vi "Main.vi"(11 "Module Admin":refnum<class "Delacor_lib_QMH_Module Admin.lvclass">) -> ()   [LabVIEW 2020, in "GUI.lvlib"]
doc: "This template is based off of the Queued Message Handler design pattern and the Queued Message Handler project template that ships with LabVIEW.\n\nThe main difference is that the queue is private to this module and communication between modules is performed via Broadcast and Request events.\n\nRequest events are wrapped in public API methods and are handled in the Event Handling Loop (EHL) of this VI. Any module can register for Broadcast events sent by this module. The EHL generates messages based on user interface actions.\n\nThe Message Handling Loop (MHL) processes messages generated by the EHL, or by other messages. The messages are string values, so new messages can be added easily to the Message Cases case structure in the MHL. Each message cluster can also provide an optional value for Message Data, which is a variant that can be converted to whatever message-specific data is required.\n_____\nBased on DQMH Project Template 6.1.0.94."
uses:
  GUI.lvlib
  <vilib>/Delacor/Delacor QMH/Libraries/Module Admin_class/Delacor_lib_QMH_Module Admin.lvclass
  <vilib>/Delacor/Delacor QMH/Libraries/Message Queue_class/Delacor_lib_QMH_Message Queue.lvclass/Delacor_lib_QMH_Message Queue.ctl
  <vilib>/Delacor/Delacor QMH/Libraries/Module Admin_class/Delacor_lib_QMH_Module Admin.lvclass/Delacor_lib_QMH_Module Admin.ctl
  <vilib>/ErrorRing/Error Ring.xnode
  <vilib>/Delacor/Delacor QMH/Libraries/Message Queue_class/Delacor_lib_QMH_Message Queue.lvclass
  Module Data--cluster.ctl
  <vilib>/Utility/miscctls.llb/LVPointTypeDef.ctl
  <vilib>/Delacor/Delacor QMH/Libraries/Message Queue_class/Delacor_lib_QMH_Enqueue Message (Single).vi
  Stop Argument--cluster.ctl
  NI DAQ/NI DAQ.lvlib
  Support/Motor parameters.ctl
  Start motor Argument--cluster.ctl
  NI DAQ/Support/Task list.ctl
  NI DAQ/Support/Continuous aquisition params.ctl
  FGV states.ctl
  Configuration/Configuration.lvlib
  Configuration/Config data.ctl
  Stop conditions.ctl
  TDS1002 Oscilloscope/TDS1002 Oscilloscope.lvlib
  Support/Channel configuration--cluster.ctl
  TDS1002 Oscilloscope/Trigger config--cluster.ctl
  Support/Motor move data.ctl
  <vilib>/Delacor/Delacor QMH/Libraries/Message Queue_class/Delacor_lib_QMH_Enqueue Message (Array).vi
  <vilib>/Utility/error.llb/Error Cluster From Error Code.vi
  Support/Stop button.ctl
  Support/Home button.ctl
  Support/Move motor.ctl
  Support/Exit button.ctl
  Support/Configure button.ctl
panel:
  out "Homing?":bool
  in  "Pasos por medición":i32=50
  out "XY Graph":cluster{"X":dbl, "Y":dbl}[](graph)
  out "Lectura del sensor":dbl format="%#_gV"
  in  "Emergency stop":T1
  in  "stop":T2
  out "current position":dbl caption="Posición actual" format="%0.4f mm"
  in  "Home Button":T3
  in  "Configure":T4
  in  "Parámetros del motor":T5={"Dirección"=enum."Avance", "Tipo"=enum."Simple", "Velocidad (RPM)"=5.0, "Cantidad de pasos"=100} {"Cantidad de pasos" min=0 max=16000 step=1; "Velocidad (RPM)" min=1.0 max=100.0 step=1.0}
  in  "Stop motor":bool
  in  "Move motor":T6
  out "error out":errorcluster
  out "Status":string caption="Estado del sistema"
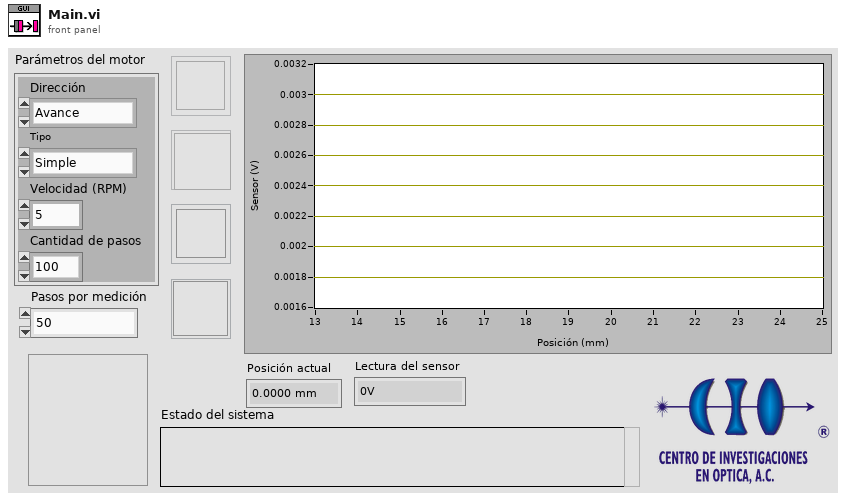
[diagram p1: front panel]
types:
  T1 = typedef "Stop button.ctl" = bool
  T2 = typedef "Exit button.ctl" = bool
  T3 = typedef "Home button.ctl" = bool
  T4 = typedef "Configure button.ctl" = bool
  T5 = cluster{"Dirección":enum16{"Avance", "Retroceso"}, "Tipo":enum16{"Simple", "Medio paso"}, "Velocidad (RPM)":dbl, "Cantidad de pasos":i32}
  T6 = typedef "Move motor.ctl" = bool
  T7 = typedef "GUI.lvlib/Module Data--cluster.ctl" = cluster{"Status":string, "DAQ mod ID":i32, "OSC mod ID":i32, "Config data":T8}
  T8 = typedef "Configuration.lvlib/Config data.ctl" = cluster{"Arduino":string, "Steps per rev":dbl, "Config path":path, "Pitch":dbl, "Osciloscopio":refnum<visa-resource-name>}
  T9 = typedef "NI DAQ.lvlib/Broadcast Events--cluster.ctl" = cluster{"Module Did Init":refnum<user-event>, "Status Updated":refnum<user-event>, "Error Reported":refnum<user-event>, "Module Did Stop":refnum<user-event>, "Update Module Execution Status":refnum<user-event>, "Digital data acquired":refnum<user-event>, "Device connected":refnum<user-event>, "Connection failed":refnum<user-event>, "Analog data acquired":refnum<user-event>, "Tasks started":refnum<user-event>}
  T10 = typedef "Configuration.lvlib/Broadcast Events--cluster.ctl" = cluster{"Module Did Init":refnum<user-event>, "Status Updated":refnum<user-event>, "Error Reported":refnum<user-event>, "Module Did Stop":refnum<user-event>, "Update Module Execution Status":refnum<user-event>}
  T11 = typedef "GUI.lvlib/Broadcast Events--cluster.ctl" = cluster{"Module Did Init":refnum<user-event>, "Status Updated":refnum<user-event>, "Error Reported":refnum<user-event>, "Module Did Stop":refnum<user-event>, "Update Module Execution Status":refnum<user-event>, "Motor stopped":refnum<user-event>}
  T12 = typedef "TDS1002 Oscilloscope.lvlib/Broadcast Events--cluster.ctl" = cluster{"Module Did Init":refnum<user-event>, "Status Updated":refnum<user-event>, "Error Reported":refnum<user-event>, "Module Did Stop":refnum<user-event>, "Update Module Execution Status":refnum<user-event>, "Helper Loop Status Updated":refnum<user-event>, "Device connected":refnum<user-event>, "Device disconnected":refnum<user-event>, "Data acquired":refnum<user-event>, "Configuration applied":refnum<user-event>}
  T13 = typedef "GUI.lvlib/Request Events--cluster.ctl" = cluster{"Stop Module":refnum<user-event>, "Show Panel":refnum<user-event>, "Hide Panel":refnum<user-event>, "Get Module Execution Status":refnum<user-event>, "Show Diagram":refnum<user-event>, "Start motor":refnum<user-event>, "Move motor":refnum<user-event>, "Stop motor":refnum<user-event>}
  T14 = typedef "Motor move data.ctl" = cluster{"current position":dbl, "Sensor reading (V)":dbl, "Home?":bool, "Steps taken":i32, "Graph data":cluster{"current position out":dbl, "Sensor reading":dbl}[], "Timeout":i32}
  T15 = typedef "GUI.lvlib/Stop conditions.ctl" = enum16{"Finish", "End-stop", "Manual"}
  T16 = cluster{"current position out":dbl, "Sensor reading":dbl}[]
  T17 = enum8{"Enabled", "Disabled", "Disabled and Grayed Out"}
  T18 = typedef "GUI.lvlib/FGV states.ctl" = enum16{"Read", "Full step", "Half step", "Release", "Reset"}
  T19 = typedef "LVPointTypeDef.ctl" = cluster{"Horizontal":i16, "Vertical":i16}
  T20 = enum32{"Invalid", "Standard", "Closed", "Hidden", "Minimized", "Maximized"}
  T21 = enum16{"All", "DO task", "DI task", "AO task", "AI task"}
  T22 = typedef "GUI.lvlib/Start motor Argument--cluster.ctl" = cluster{"Motor params":T23}
  T23 = typedef "GUI.lvlib/Motor parameters.ctl" = cluster{"Dirección":enum16{"Avance", "Retroceso"}, "Tipo":enum16{"Simple", "Medio paso"}, "Velocidad (RPM)":dbl, "Cantidad de pasos":i32, "Avance (mm)":dbl, "Pasos por rev":dbl, "Paso del tonillo":dbl}
  T24 = typedef "NI DAQ.lvlib/Task list.ctl" = enum16{"All", "DO task", "DI task", "AO task", "AI task"}
  T25 = typedef "NI DAQ.lvlib/Continuous aquisition params.ctl" = cluster{"Module ID":i32, "Task list":T24, "Timeout":i32, "Acq type":enum16{"Single", "Multiple"}, "Data in":variant, "DAQmx Task":refnum<k21>, "N samples":i32}
  T26 = typedef "GUI.lvlib/Stop Argument--cluster.ctl" = cluster{"Origin":string, "Exit via Stop Module Req?":bool, "Wait for Module to stop?":bool}
  T27 = enum32{"invalid lock state", "Not Locked", "Locked (No Password)", "Password-protected"}
  T28 = cluster{"current position":dbl, "Sensor reading (V)":dbl}
  T29 = cluster{"current position":dbl, "Sensor reading (V)":dbl}[]
  T30 = typedef "TDS1002 Oscilloscope.lvlib/Trigger config--cluster.ctl" = cluster{"Trigger Source":i32, "Trigger Mode":i32, "Trigger Slope":i32, "Trigger Coupling":i32, "Trigger Level":dbl}
  T31 = typedef "TDS1002 Oscilloscope.lvlib/Channel configuration--cluster.ctl" = cluster{"Acquisition Type":i32, "Averaged Waveforms":i32, "Channel":i32, "Probe Attenuation":i32, "Timebase":dbl}
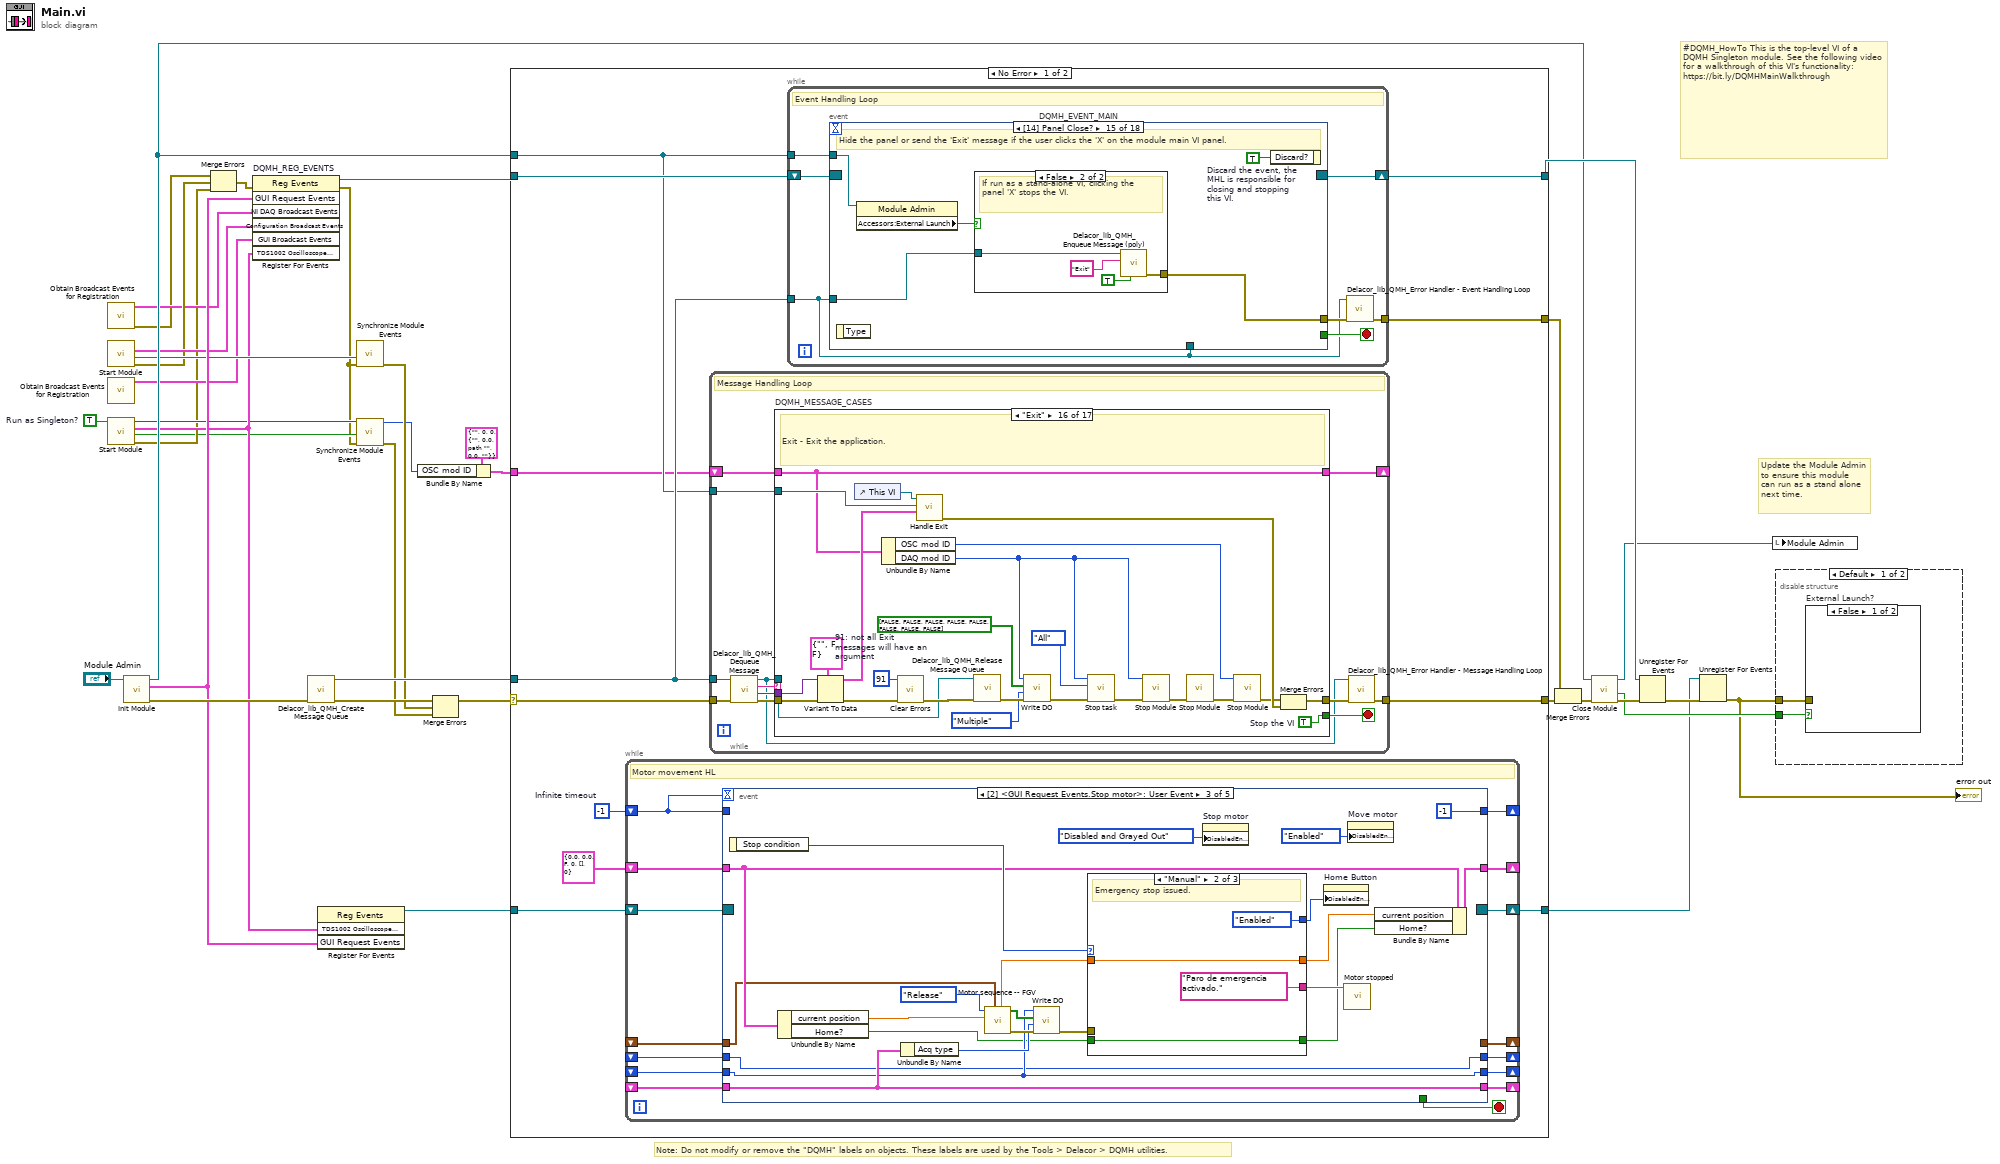
[diagram p0: block diagram]
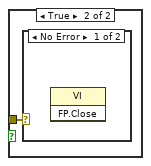
[diagram p2: hidden frame]
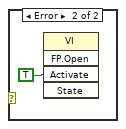
[diagram p3: hidden frame]
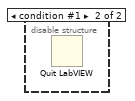
[diagram p4: hidden frame]
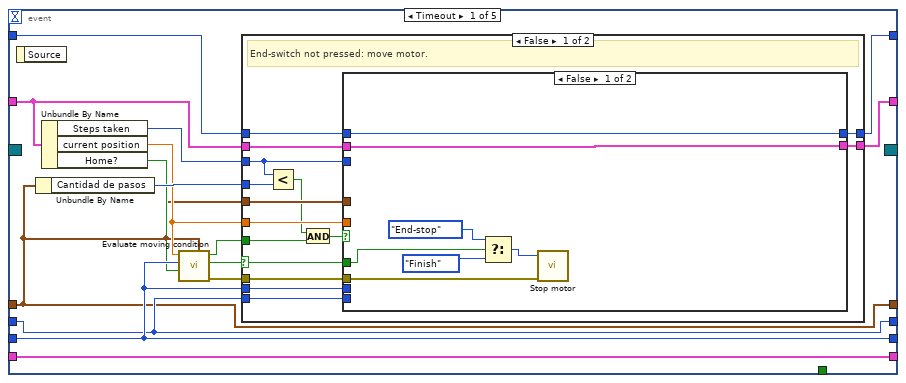
[diagram p5: hidden frame]
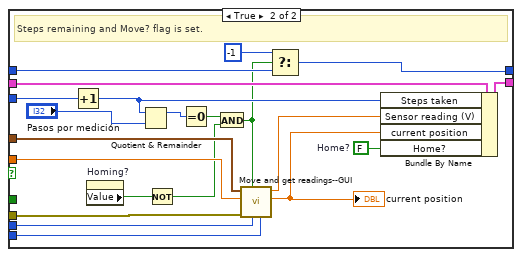
[diagram p6: hidden frame]
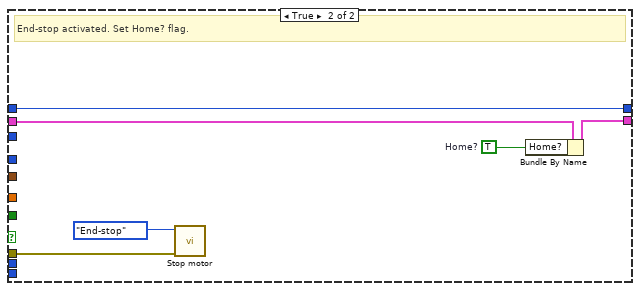
[diagram p7: hidden frame]
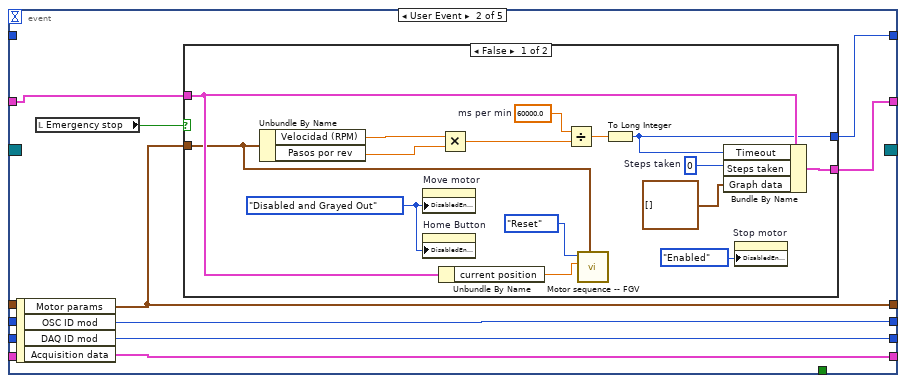
[diagram p8: hidden frame]
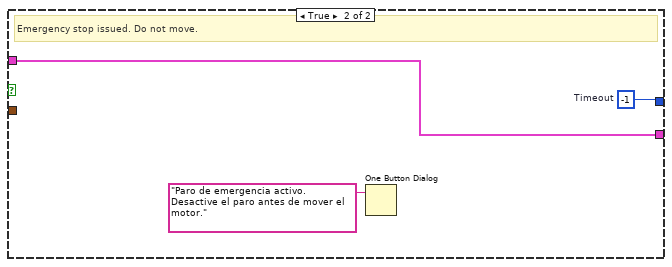
[diagram p9: hidden frame]
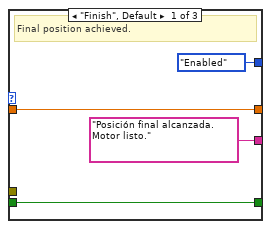
[diagram p10: hidden frame]
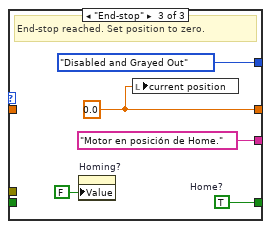
[diagram p11: hidden frame]
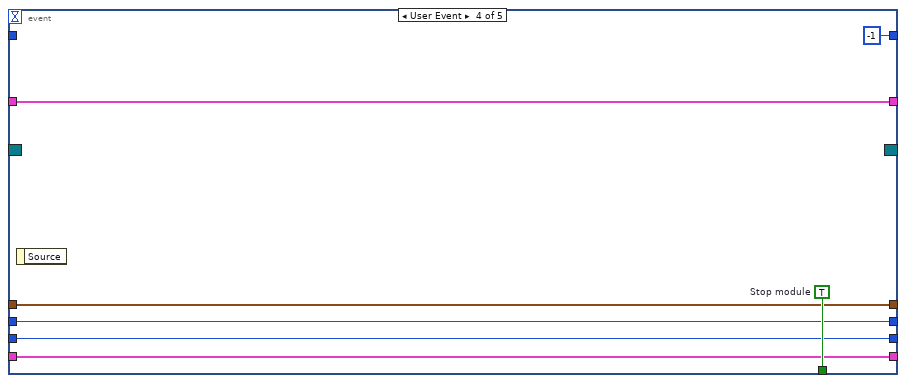
[diagram p12: hidden frame]
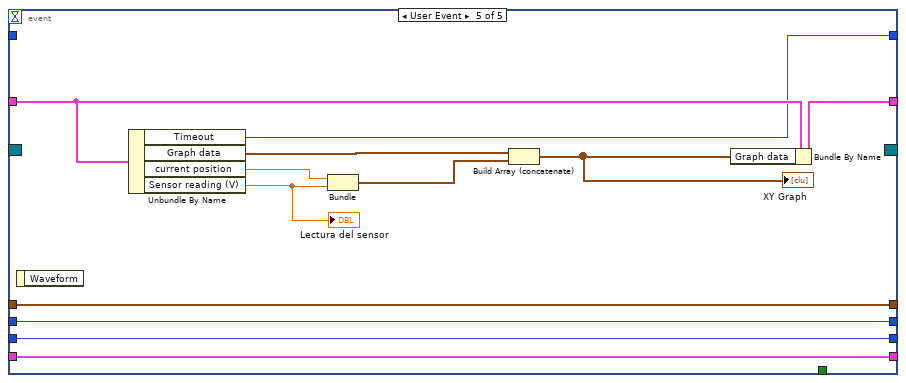
[diagram p13: hidden frame]
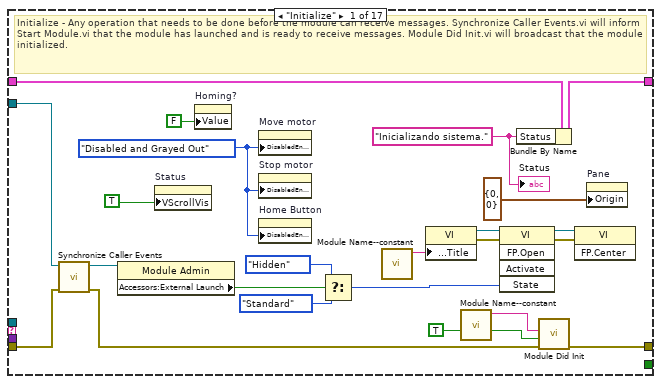
[diagram p14: hidden frame]
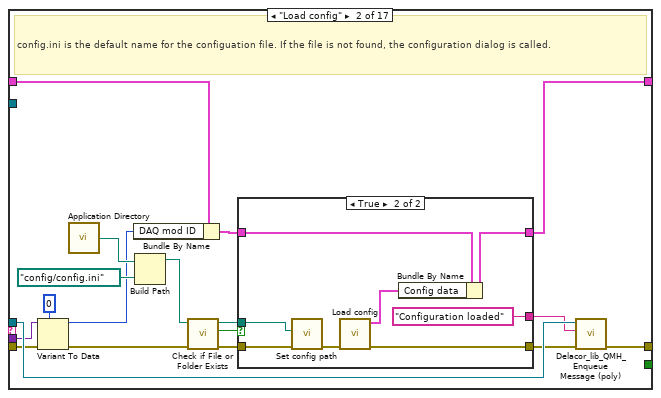
[diagram p15: hidden frame]
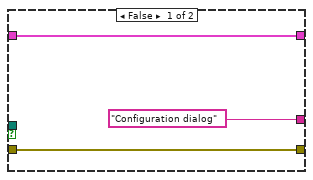
[diagram p16: hidden frame]
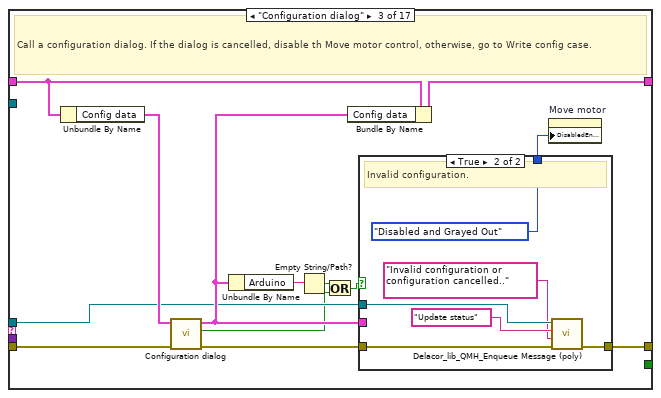
[diagram p17: hidden frame]
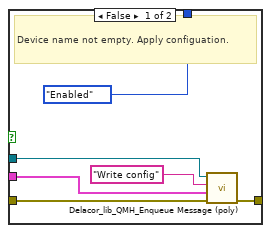
[diagram p18: hidden frame]
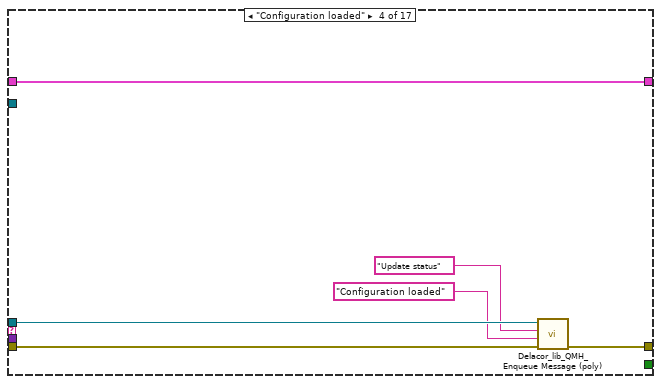
[diagram p19: hidden frame]
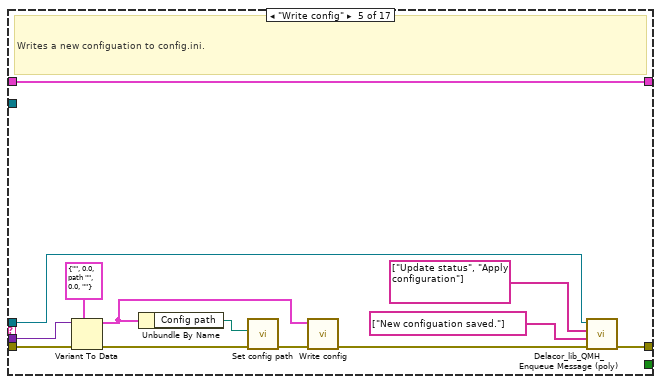
[diagram p20: hidden frame]
diagram:
  w10 = TRUE  # Run as Singleton?
  # "#DQMH_HowTo This is the top-level VI of a DQMH Singleton module. See the following video for a walkthrough of this VI's functionality: https://bit.ly/DQMHMainWalkthrough"
  # "Note: Do not modify or remove the \"DQMH\" labels on objects. These labels are used by the Tools > Delacor > DQMH utilities."
  # "Update the Module Admin to ensure this module can run as a stand alone next time."
  n1 = call "Obtain Broadcast Events for Registration.vi"() -> ("error out"=w11:errorcluster, "NI DAQ Broadcast Events"=w12:T9)  [unwired: 9 in, 1 out]
  n2 = call "Start Module.vi"() -> ("error out"=w15:errorcluster, "Wait for Event Sync?"=w18:bool, "Configuration Broadcast Events"=w17:T10)  [unwired: 8 in, 1 out]
  n3 = call "Obtain Broadcast Events for Registration.vi"() -> ("GUI Broadcast Events"=w13:T11)  [unwired: 9 in, 2 out]
  n4 = call "Start Module.vi"("Run as Singleton? (F)"=w10) -> ("error out"=w4:errorcluster, "Wait for Event Sync?"=w2:bool, "TDS1002 Oscilloscope Broadcast Events"=w9:T12, "Module ID"=w8:i32)  [unwired: 7 in]
  n5 = call "Init Module.vi"("Singleton Module Admin in"="Module Admin") -> ("error out"=w36:errorcluster, "GUI Request Events"=w24:T13, "Singleton Module Admin out"=w22:refnum<class "Delacor_lib_QMH_Module Admin.lvclass">)  [unwired: 8 in]
  n6 = Merge Errors(w11, w15, w4) -> (w16:errorcluster)
  n7 = register-events "DQMH_REG_EVENTS"(error in=w16, w24, w12, w17, w13, w9) -> (reference out=w29:refnum<event-registration>, error out=w1:errorcluster)  [unwired: 1 in]
  n8 = call <vilib>:"Delacor_lib_QMH_Create Message Queue.vi"("error in"=w36) -> ("error out"=w32:errorcluster, "Message Queue"=w28:refnum<class "Delacor_lib_QMH_Message Queue.lvclass">)  [unwired: 9 in]
  n9 = register-events(w9, w24) -> (reference out=w23:refnum<event-registration>)  [unwired: 2 in, 1 out]
  n10 = call "Synchronize Module Events.vi"("error in"=w1, "Wait for Event Sync?"=w18) -> ("error out"=w14:errorcluster)  [unwired: 9 in]
  n11 = call "Synchronize Module Events.vi"("error in"=w1, "Wait for Event Sync?"=w2, "Module ID in"=w8) -> ("error out"=w3:errorcluster, "Module ID out"=w5:i32)  [unwired: 7 in]
  n12 = Bundle By Name(cluster=T7 {"Status"="", "DAQ mod ID"=0, "OSC mod ID"=0, "Config data"={"Arduino"="", "Steps per rev"=0.0, "Config path"=path "", "Pitch"=0.0, "Osciloscopio"=""}} ("Data Cluster"), "OSC mod ID"=w5) -> (w6:T7)
  n13 = Merge Errors(w32, w14, w3) -> (w31:errorcluster)
  n14 = case shown="No Error" w31 {
    selector: w31 -> [w47 w609]
    tunnel: [w49 w608] -> w37
    tunnel: [w46 w614] -> w30
    tunnel: w29 -> [w45 w614]
    tunnel: w28 -> [w44 w607]
    tunnel: [w48 _] -> w34
    tunnel: w22 -> [w43 w610]
    tunnel: w23 -> [w40 w606]
    tunnel: [w41 w606] -> w19
    tunnel: w6 -> [w39 w604]
    frame No Error {
      w42 = -1  # Infinite timeout
      n15 = while {
        shift-right: [w60] -> _
        shift-left: w42 -> [w64]
        shift-right: [w62] -> _
        shift-left: _ -> [w61]
        shift-right: [w59] -> w41
        shift-left: w40 -> [w58]
        shift-right: [w57] -> _
        shift-left: _ -> [w56]
        shift-right: [w54] -> _
        shift-left: T14 {"current position"=0.0, "Sensor reading (V)"=0.0, "Home?"=FALSE, "Steps taken"=0, "Graph data"=[], "Timeout"=0} -> [w55]
        shift-right: [w53] -> _
        shift-left: _ -> [w52]
        shift-right: [w51] -> _
        shift-left: _ -> [w50]
        stop <- w63 stop-if-true
        # "Motor movement HL"
        n16 = event shown="[2] <GUI Request Events.Stop motor>: User Event" {
          selector: w58 -> [_ _ _ _ _]
          dyn-events: [_ _ _ _ _] -> w59
          timeout: w64 -> [_ _ _ _ _]
          tunnel: w64 -> [w67 _ _ _ _]
          tunnel: [_ _ _ w196 _] -> w63
          tunnel: [w79 w131 w168 w195 w208] -> w62
          tunnel: w61 -> [w79 _ w168 w195 w208]
          tunnel: [w66 w136 -1 -1 w198] -> w60
          tunnel: [w76 w134 w166 w193 w207] -> w57
          tunnel: w56 -> [w76 _ w166 w193 w207]
          tunnel: w55 -> [w70 w133 w160 w192 w203]
          tunnel: [w69 w132 w163 w192 w201] -> w54
          tunnel: [w68 w130 w157 w191 w199] -> w53
          tunnel: w52 -> [w68 _ w157 w191 w199]
          tunnel: [w65 w129 _ w190 w197] -> w51
          tunnel: w50 -> [w65 _ w156 w190 w197]
          event Timeout {
            n17 = event-data() -> ()  [unwired: 1 in, 1 out]
            n18 = Unbundle By Name(w65) -> ("Cantidad de pasos"=w78:i32)
            n19 = Unbundle By Name(w70) -> ("Steps taken"=w73:i32, "current position"=w72:dbl, "Home?"=w71:bool)
            n20 = call "Evaluate moving condition.vi"("Motor params"=w65, "Home?"=w71, "DAQ ID mod"=w76, "current position"=w72) -> ("error out"=w77:errorcluster, "End-stop?"=w75:bool, "Move?"=w74:bool)  [unwired: 5 in]
            n21 = case shown="False" w75 {
              selector: w75 -> [w85 _]
              tunnel: w65 -> [w94 _]
              tunnel: w73 -> [w90 _]
              tunnel: w78 -> [w93 _]
              tunnel: w77 -> [w92 w128]
              tunnel: w76 -> [w91 _]
              tunnel: w72 -> [w89 _]
              tunnel: w74 -> [w88 _]
              tunnel: w70 -> [w84 w126]
              tunnel: [w83 w124] -> w69
              tunnel: w68 -> [w82 _]
              tunnel: w67 -> [w81 w123]
              tunnel: [w80 w123] -> w66
              frame False {
                # "End-switch not pressed: move motor."
                n22 = Less?(x=w90, y=w93) -> (x < y?=w87:bool)
                n23 = And(x=w87, y=w88) -> (x .and. y?=w86:bool)
                n24 = case shown="False" w86 {
                  tunnel: w91 -> [_ w111]
                  tunnel: w94 -> [_ w120]
                  tunnel: w92 -> [w101 w122]
                  tunnel: w90 -> [_ w119]
                  tunnel: w89 -> [_ w121]
                  tunnel: w85 -> [w98 _]
                  tunnel: w84 -> [w96 w116]
                  tunnel: [w96 w115] -> w83
                  tunnel: w82 -> [_ w110]
                  tunnel: w81 -> [w95 w109]
                  tunnel: [w95 w107] -> w80
                  frame False {
                    n25 = Select(t=Stop_conditions."End-stop" ("Stop condition"), s=w98, f=Stop_conditions."Finish") -> (s? t:f=w97:T15)
                    n26 = call "Stop motor.vi"("error in"=w101, "Stop condition"=w97) -> ()  [unwired: 9 in, 1 out]
                  }
                  frame True {
                    w112 = FALSE  # Home?
                    # "Steps remaining and Move? flag is set."
                    n27 = Increment(x=w119) -> (x+1=w106:i32)
                    n28 = property on="Homing?" class="Bool (strict)"() -> ("Value"=w105:bool)  [unwired: 2 in, 2 out]
                    n29 = Quotient & Remainder(x=w106, y="Pasos por medición") -> (x-y*floor(x/y)=w117:i32)  [unwired: 1 out]
                    n30 = Not(x=w105) -> (.not. x?=w103:bool)
                    n31 = Equal To 0?(x=w117) -> (x = 0?=w104:bool)
                    n32 = And(x=w104, y=w103) -> (x .and. y?=w102:bool)
                    n33 = call "Move and get readings--GUI.vi"("OCS ID mod"=w110, "DAQ ID mod"=w111, "Read sensor?"=w102, "error in (no error)"=w122, "current position in"=w121, "Motor params"=w120) -> ("current position out"=w113:dbl, "Sensor reading"=w114:dbl)  [unwired: 3 in, 1 out]
                    "current position" <- w113
                    n34 = Select(t=-1, s=w102, f=w109) -> (s? t:f=w107:i32)
                    n35 = Bundle By Name(cluster=w116, "Steps taken"=w106, "Sensor reading (V)"=w114, "current position"=w113, "Home?"=w112) -> (w115:T14)
                  }
                }
              }
              frame True {
                w125 = TRUE  # Home?
                # "End-stop activated. Set Home? flag."
                n36 = call "Stop motor.vi"("error in"=w128, "Stop condition"=Stop_conditions."End-stop") -> ()  [unwired: 9 in, 1 out]
                n37 = Bundle By Name(cluster=w126, "Home?"=w125) -> (w124:T14)
              }
            }
          }
          event User Event {
            n38 = event-data() -> ("Motor params"=w129:T23, "OSC ID mod"=w130:i32, "DAQ ID mod"=w134:i32, "Acquisition data"=w131:T25)  [unwired: 1 in]
            n39 = local read "Emergency stop"() -> (w135:T1)
            n40 = case shown="False" w135 {
              tunnel: w129 -> [w138 _]
              tunnel: [w139 w154] -> w136
              tunnel: w133 -> [w141 w152]
              tunnel: [w143 w152] -> w132
              frame False {
                w137 = T17."Disabled and Grayed Out" ("Disabled")
                w144 = 0  # Steps taken
                w148 = 60000.0  # ms per min
                n41 = Unbundle By Name(w138) -> ("Velocidad (RPM)"=w151:dbl, "Pasos por rev"=w146:dbl)
                n42 = property on="Move motor" class="Bool"("DisabledEnum"=w137) -> ()  [unwired: 2 in, 2 out]
                n43 = property on="Home Button" class="Bool"("DisabledEnum"=w137) -> ()  [unwired: 2 in, 2 out]
                n44 = Unbundle By Name(w141) -> ("current position"=w140:dbl)
                n45 = Multiply(x=w151, y=w146) -> (x*y=w149:dbl)
                n46 = Divide(x=w148, y=w149) -> (x/y=w150:dbl)
                n47 = call "Motor sequence -- FGV.vi"("Motor params"=w138, "current position (in)"=w140, "Action"=FGV_states."Reset") -> ()  [unwired: 6 in, 3 out]
                n48 = To Long Integer(number=w150) -> (32bit integer=w139:i32)
                n49 = Bundle By Name(cluster=w141, "Timeout"=w139, "Steps taken"=w144, "Graph data"=T16 []) -> (w143:T14)
                n50 = property on="Stop motor" class="Bool"("DisabledEnum"=T17."Enabled" ("Disabled")) -> ()  [unwired: 2 in, 2 out]
              }
              frame True {
                w154 = -1  # Timeout
                # "Emergency stop issued. Do not move."
                n51 = One Button Dialog(message="Paro de emergencia activo. Desactive el paro antes de mover el motor.") -> ()  [unwired: 1 in, 1 out]
              }
            }
          }
          event User Event {
            n52 = event-data() -> ("Stop condition"=w170:T15)  [unwired: 1 in]
            n53 = Unbundle By Name(w160) -> ("current position"=w158:dbl, "Home?"=w159:bool)
            n54 = Unbundle By Name(w168) -> ("Acq type"=w173:enum16{"Single", "Multiple"})
            n55 = call "Motor sequence -- FGV.vi"("Motor params"=w156, "current position (in)"=w158, "Action"=FGV_states."Release") -> ("error out"=w175:errorcluster, "Data out"=w174:bool[], "current position (out)"=w164:dbl)  [unwired: 6 in]
            n56 = call "Write DO.vi"("error in"=w175, "Samples"=w173, "Data"=w174, "Module ID"=w166) -> ("error out"=w169:errorcluster)  [unwired: 7 in]
            n57 = case shown="\"Manual\"" w170 {
              tunnel: ["Posición final alcanzada. Motor listo." "Paro de emergencia activado." "Motor en posición de Home."] -> w167
              tunnel: w169 -> [_ _ _]
              tunnel: w164 -> [w179 w183 _]
              tunnel: [w179 w183 w188] -> w162
              tunnel: [w178 w182 w187] -> w161
              tunnel: w159 -> [w178 w182 _]
              tunnel: [T17."Enabled" ("Disabled") T17."Enabled" ("Disabled") T17."Disabled and Grayed Out" ("Disabled")] -> w155
              frame "Finish", Default {
                # "Final position achieved."
              }
              frame "Manual" {
                # "Emergency stop issued."
              }
              frame "End-stop" {
                w187 = TRUE  # Home?
                w188 = 0.0 ("current position")
                # "End-stop reached. Set position to zero."
                n58 = property on="Homing?" class="Bool (strict)"("Value"=FALSE ("Homing?")) -> ()  [unwired: 2 in, 2 out]
                n59 = local write "current position"(w188) -> ()
              }
            }
            n60 = property on="Stop motor" class="Bool"("DisabledEnum"=T17."Disabled and Grayed Out" ("Disabled")) -> ()  [unwired: 2 in, 2 out]
            n61 = property on="Home Button" class="Bool"("DisabledEnum"=w155) -> ()  [unwired: 2 in, 2 out]
            n62 = call "Motor stopped.vi"("Stop condition"=w167) -> ()  [unwired: 10 in, 1 out]
            n63 = property on="Move motor" class="Bool"("DisabledEnum"=T17."Enabled" ("Disabled")) -> ()  [unwired: 2 in, 2 out]
            n64 = Bundle By Name(cluster=w160, "current position"=w162, "Home?"=w161) -> (w163:T14)
          }
          event User Event {
            w196 = TRUE  # Stop module
            n65 = event-data() -> ()  [unwired: 1 in, 1 out]
          }
          event User Event {
            n66 = event-data() -> ()  [unwired: 1 in, 1 out]
            n67 = Unbundle By Name(w203) -> ("Timeout"=w198:i32, "Graph data"=w204:T16, "current position"=w206:dbl, "Sensor reading (V)"=w200:dbl)
            "Lectura del sensor" <- w200
            n68 = Bundle("current position"=w206, "Sensor reading (V)"=w200) -> (w205:T28)  [unwired: 1 in]
            n69 = Build Array (concatenate)(w204, w205) -> (w202:T29)
            "XY Graph" <- w202
            n70 = Bundle By Name(cluster=w203, "Graph data"=w202) -> (w201:T14)
          }
        }
      }
      n71 = while {
        tunnel: w44 -> [w211]
        shift-right: [w215] -> _
        shift-left: w39 -> [w216]
        tunnel: w47 -> [w219]
        tunnel: [w217] -> w49
        tunnel: w43 -> [w209]
        stop <- w214 stop-if-true
        # "Message Handling Loop"
        n72 = call-dynamic "Delacor_lib_QMH_Dequeue Message.vi"("error in"=w219, "Message Queue in"=w211) -> ("error out"=w218:errorcluster, "Message Data"=w212:variant, "Message"=w213:string, "Message Queue out"=w210:refnum<class "Delacor_lib_QMH_Message Queue.lvclass">)  [unwired: 6 in]
        n73 = case "DQMH_MESSAGE_CASES" shown="\"Exit\"" w213 {
          selector: w213 -> [_ _ _ _ _ _ _ _ _ _ _ _ _ _ _ _ w489]
          tunnel: w210 -> [_ w254 w276 w300 w306 w322 w332 w344 _ _ w395 w417 w432 _ w449 w482 _]
          tunnel: w218 -> [w241 w250 w285 w302 w314 w326 w329 w348 w374 w382 w401 w423 w431 w446 w456 w487 w491]
          tunnel: [w239 w252 w280 w301 w307 w323 w333 w349 w363 w376 w398 w420 w433 w446 w452 w485 w492] -> w220
          tunnel: w216 -> [w224 w246 w283 w303 w316 w325 w327 w350 w367 w379 w404 w426 w434 w445 w451 w474 w490]
          tunnel: [w230 w255 w282 w303 w316 w325 w327 w350 w366 w379 w404 w426 w434 w445 w451 w474 w490] -> w215
          tunnel: [_ _ _ _ _ _ _ _ _ _ _ _ _ _ _ w481 _] -> w214
          tunnel: w212 -> [_ w248 _ _ w312 _ _ _ w373 w381 _ _ w429 _ w450 w480 _]
          tunnel: w209 -> [w231 _ _ _ _ _ _ _ _ _ _ _ _ _ w448 w475 _]
          frame "Initialize" {
            w221 = T17."Disabled and Grayed Out" ("Disabled")
            w226 = "Inicializando sistema." ("Initial Message")
            # "Initialize - Any operation that needs to be done before the module can receive messages. Synchronize Caller Events.vi will inform Start Module.vi that the module has launched and is ready to receive messages. Module Did Init.vi will broadcast that the module initialized."
            n74 = call "Synchronize Caller Events.vi"("error in (no error)"=w241, "Singleton Module Admin in"=w231) -> ("error out"=w240:errorcluster, "Singleton Module Admin out"=w227:refnum<class "Delacor_lib_QMH_Module Admin.lvclass">)  [unwired: 8 in]
            n75 = property class="Module Admin"(reference=w227) -> ("Accessors:External Launch"=w235:bool)  [unwired: 1 in, 2 out]
            n76 = property on="Status" class="Str"("VScrollVis"=TRUE ("Horizontal Scrollbar Visible")) -> ()  [unwired: 2 in, 2 out]
            n77 = property on="Homing?" class="Bool (strict)"("Value"=FALSE ("Homing?")) -> ()  [unwired: 2 in, 2 out]
            n78 = property on="Move motor" class="Bool"("DisabledEnum"=w221) -> ()  [unwired: 2 in, 2 out]
            n79 = property on="Stop motor" class="Bool"("DisabledEnum"=w221) -> ()  [unwired: 2 in, 2 out]
            n80 = property on="Home Button" class="Bool"("DisabledEnum"=w221) -> ()  [unwired: 2 in, 2 out]
            n81 = Select(t=T20."Hidden" ("State"), s=w235, f=T20."Standard" ("State")) -> (s? t:f=w232:T20)
            n82 = call "Module Name--constant.vi"() -> ("Module Name"=w238:string)  [unwired: 11 in]
            n83 = property class="VI"("Front Panel.Title"=w238) -> (reference out=w237:refnum<vi>, error out=w243:errorcluster)  [unwired: 2 in]
            n84 = call "Module Name--constant.vi"() -> ("Module Name"=w228:string)  [unwired: 11 in]
            n85 = invoke class="VI" method="FP.Open"(reference=w237, error in=w243, "State"=w232) -> (reference out=w236:refnum<vi>, error out=w242:errorcluster)  [unwired: 2 in, 3 out]
            n86 = Bundle By Name(cluster=w224, "Status"=w226) -> (w230:T7)
            n87 = call "Module Did Init.vi"("error in (no error)"=w240, "Initialized?"=TRUE, "Origin"=w228) -> ("error out"=w239:errorcluster)  [unwired: 8 in]
            n88 = invoke class="VI" method="FP.Center"(reference=w236, error in=w242) -> ()  [unwired: 1 in, 3 out]
            n89 = property on="Pane" class="Pane"("Origin"=T19 {"Horizontal"=0, "Vertical"=0}) -> ()  [unwired: 2 in, 2 out]
            "Status" <- w226
          }
          frame "Load config" {
            # "config.ini is the default name for the configuation file. If the file is not found, the configuration dialog is called."
            n90 = Variant To Data(error in=w250, type=0 ("Module ID out"), Variant=w248) -> (data=w244:i32, error out=w249:errorcluster)
            n91 = call <vilib>:"Application Directory.vi"() -> ("Application Directory"=w261:path)
            n92 = Bundle By Name(cluster=w246, "DAQ mod ID"=w244) -> (w245:T7)
            n93 = Build Path(base path=w261, name or relative path=path "config/config.ini") -> (appended path=w259:path)
            n94 = call <vilib>:"Check if File or Folder Exists.vi"("error in (no error)"=w249, "path"=w259) -> ("error out"=w258:errorcluster, "file or folder exists?"=w257:bool, "dup path"=w256:path)  [unwired: 7 in]
            n95 = case shown="True" w257 {
              tunnel: w258 -> [w262 w267]
              tunnel: w256 -> [_ w265]
              tunnel: w245 -> [w264 w272]
              tunnel: [w264 w270] -> w255
              tunnel: [w262 w269] -> w253
              tunnel: ["Configuration dialog" "Configuration loaded"] -> w251
              frame False {
              }
              frame True {
                n96 = call "Set config path.vi"("error in"=w267, "Config path"=w265) -> ("error out"=w266:errorcluster)  [unwired: 9 in]
                n97 = call "Load config.vi"("error in"=w266) -> ("error out"=w269:errorcluster, "Config data"=w271:T8)  [unwired: 8 in, 1 out]
                n98 = Bundle By Name(cluster=w272, "Config data"=w271) -> (w270:T7)
              }
            }
            n99 = call-poly <vilib>:"Delacor_lib_QMH_Enqueue Message (poly).vi"("error in"=w253, "Message"=w251, "Message Queue in"=w254) -> ("error out"=w252:errorcluster)  [unwired: 7 in, 1 out]
          }
          frame "Configuration dialog" {
            # "Call a configuration dialog. If the dialog is cancelled, disable th Move motor control, otherwise, go to Write config case."
            n100 = Unbundle By Name(w283) -> ("Config data"=w284:T8)
            n101 = call "Configuration dialog.vi"("error in (no error)"=w285, "Data in"=w284) -> ("error out"=w281:errorcluster, "Cancelled?"=w273:bool, "Data out"=w277:T8)  [unwired: 7 in]
            n102 = Unbundle By Name(w277) -> ("Arduino"=w279:string)
            n103 = Empty String/Path?(string/path=w279) -> (empty?=w278:bool)
            n104 = Or(x=w278, y=w273) -> (x .or. y?=w274:bool)
            n105 = Bundle By Name(cluster=w283, "Config data"=w277) -> (w282:T7)
            n106 = case shown="True" w274 {
              tunnel: w281 -> [w290 w296]
              tunnel: [w291 w297] -> w280
              tunnel: w277 -> [w286 _]
              tunnel: w276 -> [w289 w295]
              tunnel: [T17."Enabled" ("Disabled") T17."Disabled and Grayed Out" ("Disabled")] -> w275
              frame False {
                # "Device name not empty. Apply configuation."
                n107 = call-poly <vilib>:"Delacor_lib_QMH_Enqueue Message (poly).vi"("error in"=w290, "Message Data"=w286, "Message"="Write config", "Message Queue in"=w289) -> ("error out"=w291:errorcluster)  [unwired: 6 in, 1 out]
              }
              frame True {
                # "Invalid configuration."
                n108 = call-poly <vilib>:"Delacor_lib_QMH_Enqueue Message (poly).vi"("error in"=w296, "Message Data"="Invalid configuration or configuration cancelled.." ("Message"), "Message"="Update status", "Message Queue in"=w295) -> ("error out"=w297:errorcluster)  [unwired: 6 in, 1 out]
              }
            }
            n109 = property on="Move motor" class="Bool"("DisabledEnum"=w275) -> ()  [unwired: 2 in, 2 out]
          }
          frame "Configuration loaded" {
            n110 = call-poly <vilib>:"Delacor_lib_QMH_Enqueue Message (poly).vi"("error in"=w302, "Message Data"="Configuration loaded" ("Message"), "Message"="Update status", "Message Queue in"=w300) -> ("error out"=w301:errorcluster)  [unwired: 6 in, 1 out]
          }
          frame "Write config" {
            # "Writes a new configuation to config.ini."
            n111 = Variant To Data(error in=w314, type=T8 {"Arduino"="", "Steps per rev"=0.0, "Config path"=path "", "Pitch"=0.0, "Osciloscopio"=""} ("Data"), Variant=w312) -> (data=w310:T8, error out=w313:errorcluster)
            n112 = Unbundle By Name(w310) -> ("Config path"=w309:path)
            n113 = call "Set config path.vi"("error in"=w313, "Config path"=w309) -> ("error out"=w315:errorcluster)  [unwired: 9 in]
            n114 = call "Write config.vi"("error in"=w315, "Data"=w310) -> ("error out"=w308:errorcluster)  [unwired: 9 in]
            n115 = call-poly <vilib>:"Delacor_lib_QMH_Enqueue Message (poly).vi"("error in"=w308, "Message Data Array"=string[] ["New configuation saved."] ("Message"), "Message Array"=string[] ["Update status", "Apply configuration"] ("Message"), "Message Queue in"=w306) -> ("error out"=w307:errorcluster)  [unwired: 6 in, 1 out]
          }
          frame "Apply configuration" {
            n116 = Unbundle By Name(w325) -> ("DAQ mod ID"=w319:i32, "OSC mod ID"=w324:i32)
            n117 = call "Disconnect.vi"("error in"=w326, "Module ID"=w324) -> ("error out"=w320:errorcluster)  [unwired: 9 in]
            n118 = call "Delete task.vi"("error in"=w320, "Task to stop/delete"=T21."All", "Module ID"=w319) -> ("error out"=w317:errorcluster)  [unwired: 8 in]
            n119 = call-poly <vilib>:"Delacor_lib_QMH_Enqueue Message (poly).vi"("error in"=w317, "Message Array"=string[] ["Configure oscilloscope", "Create motor task"], "Message Queue in"=w322) -> ("error out"=w323:errorcluster)  [unwired: 7 in, 1 out]
          }
          frame "Create motor task" {
            # "Create a task to output to lines 0 to 3 on the device found in config.ini"
            n120 = Unbundle By Name(w327) -> ("DAQ mod ID"=w328:i32, "Config data.Arduino"=w330:string)
            n121 = call "Create DAQ tasks--GUI.vi"("error in (no error)"=w329, "Device name"=w330, "DAQ mod ID"=w328) -> ("error out"=w331:errorcluster)  [unwired: 8 in]
            n122 = case shown="No Error" w331 {
              selector: w331 -> [w334 w343]
              tunnel: [w338 w342] -> w333
              tunnel: w332 -> [w336 w341]
              frame No Error {
                n123 = call-poly <vilib>:"Delacor_lib_QMH_Enqueue Message (poly).vi"("error in"=w334, "Message Data Array"=string[] ["Motor ready. Standing by..."] ("Status"), "Message Array"=string[] ["Update status", "Configure oscilloscope"] ("Message"), "Message Queue in"=w336) -> ("error out"=w338:errorcluster)  [unwired: 6 in, 1 out]
              }
              frame Error {
                n124 = call <vilib>:"Clear Errors.vi"("error in (no error)"=w343) -> ("error out"=w339:errorcluster)  [unwired: 5 in, 1 out]
                n125 = call-poly <vilib>:"Delacor_lib_QMH_Enqueue Message (poly).vi"("error in"=w339, "Message"="Configuration dialog", "Message Queue in"=w341) -> ("error out"=w342:errorcluster)  [unwired: 7 in, 1 out]
              }
            }
          }
          frame "Configure oscilloscope" {
            n126 = Unbundle By Name(w350) -> ("OSC mod ID"=w346:i32, "Config data.Osciloscopio"=w345:refnum<visa-resource-name>)
            n127 = call "Connect.vi"("error in"=w348, "VISA resource name"=w345, "Module ID"=w346) -> ("error out"=w347:errorcluster)  [unwired: 8 in]
            n128 = case shown="No Error" w347 {
              selector: w347 -> [w352 w358]
              tunnel: [w355 w361] -> w349
              tunnel: w346 -> [w351 _]
              tunnel: w344 -> [_ w360]
              frame No Error {
                w353 = T30 {"Trigger Source"=0, "Trigger Mode"=0, "Trigger Slope"=0, "Trigger Coupling"=1, "Trigger Level"=0.0}  # Trigger config
                w354 = T31 {"Acquisition Type"=0, "Averaged Waveforms"=4, "Channel"=0, "Probe Attenuation"=1, "Timebase"=0.0005}  # Config parameters
                n129 = call "Configure acquisition.vi"("Config parameters"=w354, "error in"=w352, "Type"=enum16{"On demand", "Continous"}."Continous", "Module ID"=w351) -> ("error out"=w355:errorcluster)  [unwired: 7 in]
                n130 = call "Configure trigger.vi"("Trigger config"=w353, "Module ID"=w351) -> ()  [unwired: 9 in, 1 out]
              }
              frame Error {
                n131 = call <vilib>:"Clear Errors.vi"("error in (no error)"=w358) -> ("error out"=w357:errorcluster)  [unwired: 5 in, 1 out]
                n132 = call-poly <vilib>:"Delacor_lib_QMH_Enqueue Message (poly).vi"("error in"=w357, "Message"="Configuration dialog", "Message Queue in"=w360) -> ("error out"=w361:errorcluster)  [unwired: 7 in, 1 out]
              }
            }
          }
          frame "Update status" {
            n133 = Variant To Data(error in=w374, type="", Variant=w373) -> (data=w370:string, error out=w364:errorcluster)
            n134 = Unbundle By Name(w367) -> ("Status"=w369:string)
            n135 = Format Into String(format string="\\n%s", w370) -> (resulting string=w368:string)  [unwired: 2 in, 1 out]
            n136 = Concatenate Strings(w369, w368) -> (w362:string)
            n137 = Bundle By Name(cluster=w367, "Status"=w362) -> (w366:T7)
            n138 = property on="Status" class="Str"(error in=w364, "Value"=w362, "Text.Scroll Position"=u32 1000) -> (error out=w363:errorcluster)  [unwired: 1 in, 1 out]
          }
          frame "Start motor" {
            # "Request to start a motor given is input parameters.\nUnused"
            n139 = Unbundle By Name(w379) -> ("DAQ mod ID"=w375:i32)
            n140 = Variant To Data(error in=w382, type=T22 {"Motor params"={"Dirección"=enum."Avance", "Tipo"=enum."Simple", "Velocidad (RPM)"=5.0, "Cantidad de pasos"=1, "Avance (mm)"=0.0, "Pasos por rev"=200.0, "Paso del tonillo"=0.0}} ("Start motor Argument"), Variant=w381) -> (data=w378:T22, error out=w377:errorcluster)
            n141 = Unbundle By Name(w378) -> ()  [unwired: 2 out]
            n142 = call "Start task.vi"("error in"=w377, "Module ID"=w375) -> ("error out"=w376:errorcluster)  [unwired: 9 in]
          }
          frame "Move motor" {
            n143 = Unbundle By Name(w404) -> ("DAQ mod ID"=w386:i32, "OSC mod ID"=w384:i32, "Config data.Pitch"=w387:dbl, "Config data.Steps per rev"=w388:dbl)
            n144 = Unbundle By Name("Parámetros del motor") -> ("Dirección"=w389:enum16{"Avance", "Retroceso"}, "Tipo"=w392:enum16{"Simple", "Medio paso"}, "Velocidad (RPM)"=w391:dbl, "Cantidad de pasos"=w390:i32)
            n145 = Bundle By Name(cluster=T23 {"Dirección"=enum."Avance", "Tipo"=enum."Simple", "Velocidad (RPM)"=30.0, "Cantidad de pasos"=1000, "Avance (mm)"=0.0, "Pasos por rev"=200.0, "Paso del tonillo"=0.0} ("Motor parameters"), "Paso del tonillo"=w387, "Pasos por rev"=w388, "Dirección"=w389, "Tipo"=w392, "Velocidad (RPM)"=w391, "Cantidad de pasos"=w390) -> (w383:T23)
            n146 = Bundle By Name(cluster=T25 {"Module ID"=0, "Task list"=enum."All", "Timeout"=0, "Acq type"=enum."Single", "Data in"=variant, "DAQmx Task"="", "N samples"=0} ("Acquisition data"), "Task list"=Task_list."DO task", "Acq type"=enum16{"Single", "Multiple"}."Multiple" ("Samples")) -> (w385:T25)
            n147 = call "Move motor.vi"("Motor params"=w383, "error in"=w401, "Acquisition data"=w385, "OSC ID mod"=w384, "DAQ ID mod"=w386) -> ("error out"=w399:errorcluster)  [unwired: 6 in]
            n148 = call-poly <vilib>:"Delacor_lib_QMH_Enqueue Message (poly).vi"("error in"=w399, "Message Data"="Motor started." ("Status"), "Message"="Update status", "Message Queue in"=w395) -> ("error out"=w398:errorcluster)  [unwired: 6 in, 1 out]
          }
          frame "Home" {
            n149 = Unbundle By Name(w426) -> ("DAQ mod ID"=w409:i32, "OSC mod ID"=w408:i32, "Config data.Pitch"=w410:dbl, "Config data.Steps per rev"=w415:dbl)
            n150 = Bundle By Name(cluster=T23 {"Dirección"=enum."Avance", "Tipo"=enum."Simple", "Velocidad (RPM)"=30.0, "Cantidad de pasos"=1000, "Avance (mm)"=0.0, "Pasos por rev"=200.0, "Paso del tonillo"=0.0} ("Motor parameters"), "Paso del tonillo"=w410, "Pasos por rev"=w415, "Dirección"=enum16{"Avance", "Retroceso"}."Retroceso", "Tipo"=enum16{"Simple", "Medio paso"}."Simple", "Velocidad (RPM)"=30.0, "Cantidad de pasos"=16000) -> (w405:T23)
            n151 = Bundle By Name(cluster=T25 {"Module ID"=0, "Task list"=enum."All", "Timeout"=0, "Acq type"=enum."Single", "Data in"=variant, "DAQmx Task"="", "N samples"=0} ("Acquisition data"), "Task list"=Task_list."DO task", "Acq type"=enum16{"Single", "Multiple"}."Multiple" ("Samples")) -> (w407:T25)
            n152 = call "Move motor.vi"("Motor params"=w405, "error in"=w423, "Acquisition data"=w407, "OSC ID mod"=w408, "DAQ ID mod"=w409) -> ("error out"=w421:errorcluster)  [unwired: 6 in]
            n153 = call-poly <vilib>:"Delacor_lib_QMH_Enqueue Message (poly).vi"("error in"=w421, "Message Data"="Homing." ("Status"), "Message"="Update status", "Message Queue in"=w417) -> ("error out"=w420:errorcluster)  [unwired: 6 in, 1 out]
            "Homing?" <- TRUE ("Homing?")
          }
          frame "Stop motor" {
            n154 = Variant To Data(error in=w431, type=TRUE, Variant=w429) -> (data=w428:bool, error out=w430:errorcluster)
            n155 = case shown="True" w428 {
              tunnel: [w436 w444] -> w433
              tunnel: w432 -> [_ w440]
              tunnel: w430 -> [w436 w438]
              frame False {
                # "Emergency stop released"
                n156 = property on="Move motor" class="Bool"("DisabledEnum"=T17."Enabled" ("Disabled")) -> ()  [unwired: 2 in, 2 out]
              }
              frame True {
                w437 = T17."Disabled and Grayed Out" ("Disabled")
                # "Emergency stop issued"
                n157 = call "Stop motor.vi"("error in"=w438, "Stop condition"=Stop_conditions."Manual") -> ("error out"=w443:errorcluster)  [unwired: 9 in]
                n158 = property on="Move motor" class="Bool"("DisabledEnum"=w437) -> ()  [unwired: 2 in, 2 out]
                n159 = property on="Stop motor" class="Bool"("DisabledEnum"=w437) -> ()  [unwired: 2 in, 2 out]
                n160 = call-poly <vilib>:"Delacor_lib_QMH_Enqueue Message (poly).vi"("error in"=w443, "Message Data"="Motor stopped." ("Status"), "Message"="Update status", "Message Queue in"=w440) -> ("error out"=w444:errorcluster)  [unwired: 6 in, 1 out]
              }
            }
          }
          frame "---Exit and Error Handling---" {
            # "Separator - The following cases handle errors and exit messages."
          }
          frame "Error" {
            # "#CodeRecommended - If you ever change the name of this \"Error\" message, you'll need to update the name in the Check Loop Error.vi as well."
            # "#CodeRecommended - If the module is running in standalone mode (External Launch = FALSE), this code will pop up an error dialog and call the 'Exit' message if an error occurs. Add more fine-grained error handling here."
            # "Error - Check the error message data and respond accordingly. This message is sent by the \"Error Handler\" VIs at the end of each loop in this application."
            n161 = property class="Module Admin"(reference=w448) -> ("Accessors:External Launch"=w447:bool)  [unwired: 1 in, 2 out]
            n162 = Variant To Data(error in=w456, type=errorcluster {"status"=FALSE, "code"=0, "source"=""} ("error constant"), Variant=w450) -> (data=w457:errorcluster, error out=w454:errorcluster)
            n163 = call "Error Reported.vi"("Error"=w457) -> ()  [unwired: 10 in, 1 out]
            n164 = case shown="False" w447 {
              tunnel: [w462 _] -> w453
              tunnel: w449 -> [w460 _]
              tunnel: w457 -> [w461 _]
              frame False {
                # "If the module is running standalone, then pop up an error dialog and call the \"Exit\" message."
                n165 = call <vilib>:"Simple Error Handler.vi"("error in (no error)"=w461) -> ()  [unwired: 4 in, 5 out]
                n166 = call-poly <vilib>:"Delacor_lib_QMH_Enqueue Message (poly).vi"("Priority Message? (F)"=TRUE, "Message"="Exit", "Message Queue in"=w460) -> ("error out"=w462:errorcluster)  [unwired: 7 in, 1 out]
              }
              frame True {
                # "If the module was launched externally, calling the Error Reported broadcast VI is the only action performed by the \"Error\" message. The module's caller can then process the error appropriately."
              }
            }
            n167 = Merge Errors(w454, w453) -> (w452:errorcluster)
            n168 = local write "error out"(w452) -> ()
          }
          frame "Exit" {
            w479 = 91  # 91: not all Exit messages will have an argument
            w481 = TRUE  # Stop the VI
            # "Exit - Exit the application."
            n169 = Variant To Data(error in=w487, type=T26 {"Origin"="", "Exit via Stop Module Req?"=FALSE, "Wait for Module to stop?"=FALSE} ("Stop Argument"), Variant=w480) -> (data=w477:T26, error out=w484:errorcluster)
            n170 = control-ref of="This VI"() -> (w476:refnum<vi>)
            n171 = Unbundle By Name(w474) -> ("OSC mod ID"=w468:i32, "DAQ mod ID"=w465:i32)
            n172 = call <vilib>:"Clear Errors.vi"("error in (no error)"=w484, "specific error code to clear (0: all)"=w479) -> ("error out"=w486:errorcluster)  [unwired: 4 in, 1 out]
            n173 = call "Handle Exit.vi"("Stop Argument"=w477, "Admin in"=w475, "VI reference"=w476) -> ("error out"=w483:errorcluster)  [unwired: 7 in, 1 out]
            n174 = call-dynamic "Delacor_lib_QMH_Release Message Queue.vi"("error in"=w486, "Message Queue"=w482) -> ("error out"=w467:errorcluster)  [unwired: 9 in]
            n175 = call "Write DO.vi"("error in"=w467, "Samples"=enum16{"Single", "Multiple"}."Multiple", "Data"=bool[] [FALSE, FALSE, FALSE, FALSE, FALSE, FALSE, FALSE, FALSE], "Module ID"=w465) -> ("error out"=w466:errorcluster)  [unwired: 7 in]
            n176 = call "Stop task.vi"("error in"=w466, "Task list"=T21."All", "Module ID"=w465) -> ("error out"=w472:errorcluster)  [unwired: 8 in]
            n177 = call "Stop Module.vi"("error in"=w472, "Module ID"=w465) -> ("error out"=w471:errorcluster)  [unwired: 9 in]
            n178 = call "Stop Module.vi"("error in"=w471) -> ("error out"=w470:errorcluster)  [unwired: 10 in]
            n179 = call "Stop Module.vi"("error in"=w470, "Module ID"=w468) -> ("error out"=w469:errorcluster)  [unwired: 9 in]
            n180 = Merge Errors(w469, w483) -> (w485:errorcluster)
          }
          frame Default {
            # "'Default' case only runs if there is a message that isn't defined in any of the other cases.  Output a programming error."
            n181 = call "Module Name--constant.vi"() -> ("Module Name"=w488:string)  [unwired: 11 in]
            n182 = xnode "Error Ring"("parameter 0"=w489, "parameter 1"=w488) -> ("error out"=w493:errorcluster)
            n183 = Merge Errors(w491, w493) -> (w492:errorcluster)
          }
        }
        n184 = call-dynamic "Delacor_lib_QMH_Error Handler - Message Handling Loop.vi"("error in"=w220, "Message Queue in"=w210) -> ("dup error in"=w217:errorcluster)  [unwired: 8 in, 1 out]
      }
      n185 = while {
        tunnel: w44 -> [w502]
        shift-right: [w505] -> w46
        shift-left: w45 -> [w506]
        tunnel: [w507] -> w48
        tunnel: w43 -> [w503]
        stop <- w504 stop-if-true
        # "Event Handling Loop"
        n186 = event "DQMH_EVENT_MAIN" shown="[14] Panel Close?" {
          selector: w506 -> [w512 _ _ _ _ _ _ _ _ _ _ _ _ _ _ _ _ _]
          dyn-events: [w511 _ _ _ _ _ _ _ _ _ _ _ _ _ _ _ _ _] -> w505
          timeout: _ -> [_ _ _ _ _ _ _ _ _ _ _ _ _ _ _ _ _ _]
          tunnel: [_ _ _ _ _ _ _ _ _ _ _ _ TRUE ("Discard?") _ _ _ _ _] -> w504
          tunnel: w502 -> [w520 w523 w525 w533 _ w541 w544 w551 _ _ _ _ w574 w581 w585 w594 w598 w601]
          tunnel: [w521 w524 w526 w534 w537 w542 w545 w546 _ _ w557 _ w577 w582 w587 w595 w599 w602] -> w508
          tunnel: w503 -> [_ _ _ _ _ _ _ _ _ _ _ _ _ _ w584 _ _ _]
          tunnel: w502 -> [_ _ _ _ w538 _ _ _ _ _ _ _ _ _ _ _ _ _]
          event User Event {
            w518 = TRUE  # Run as Singleton?
            n187 = event-data() -> ()  [unwired: 1 in, 1 out]
            n188 = call "Start Module.vi"("Run as Singleton? (F)"=w518) -> ("error out"=w515:errorcluster, "Wait for Event Sync?"=w510:bool, "NI DAQ Broadcast Events"=w514:T9, "Module ID"=w517:i32)  [unwired: 7 in]
            n189 = register-events(reference=w512, error in=w515, w514) -> (reference out=w511:refnum<event-registration>, error out=w513:errorcluster)  [unwired: 4 in]
            n190 = call "Synchronize Module Events.vi"("error in"=w513, "Wait for Event Sync?"=w510, "Module ID in"=w517) -> ("error out"=w516:errorcluster, "Module ID out"=w509:i32)  [unwired: 7 in]
            n191 = call-poly <vilib>:"Delacor_lib_QMH_Enqueue Message (poly).vi"("error in"=w516, "Message Data"=w509, "Message"="Load config", "Message Queue in"=w520) -> ("error out"=w521:errorcluster)  [unwired: 6 in, 1 out]
          }
          event User Event {
            n192 = event-data() -> ()  [unwired: 1 in, 1 out]
            n193 = call-poly <vilib>:"Delacor_lib_QMH_Enqueue Message (poly).vi"("Message"="Create motor task", "Message Queue in"=w523) -> ("error out"=w524:errorcluster)  [unwired: 8 in, 1 out]
          }
          event User Event {
            n194 = event-data() -> ()  [unwired: 1 in, 1 out]
            n195 = disable-structure shown="Disabled" {
              disable-tunnel: [w529 _] -> w526
              disable-tunnel: w525 -> [w528 _]
              frame Disabled {
                n196 = call-poly <vilib>:"Delacor_lib_QMH_Enqueue Message (poly).vi"("Message"="Configure oscilloscope", "Message Queue in"=w528) -> ("error out"=w529:errorcluster)  [unwired: 8 in, 1 out]
              }
              frame Enabled {
              }
            }
          }
          event User Event {
            w530 = T17."Enabled" ("Disabled")
            n197 = event-data() -> ()  [unwired: 1 in, 1 out]
            n198 = property on="Home Button" class="Bool"("DisabledEnum"=w530) -> ()  [unwired: 2 in, 2 out]
            n199 = property on="Move motor" class="Bool"("DisabledEnum"=w530) -> ()  [unwired: 2 in, 2 out]
            n200 = call-poly <vilib>:"Delacor_lib_QMH_Enqueue Message (poly).vi"("Message Data"="All devices ready." ("Message"), "Message"="Update status", "Message Queue in"=w533) -> ("error out"=w534:errorcluster)  [unwired: 7 in, 1 out]
          }
          event User Event {
            n201 = event-data() -> ("Error"=w539:errorcluster)  [unwired: 1 in]
            n202 = call <vilib>:"Clear Errors.vi"("error in (no error)"=w539) -> ("error out"=w536:errorcluster)  [unwired: 5 in, 1 out]
            n203 = call-poly <vilib>:"Delacor_lib_QMH_Enqueue Message (poly).vi"("error in"=w536, "Message"="Configuration dialog", "Message Queue in"=w538) -> ("error out"=w537:errorcluster)  [unwired: 7 in, 1 out]
          }
          event Value Change {
            n204 = event-data() -> ()  [unwired: 1 in, 1 out]
            n205 = call-poly <vilib>:"Delacor_lib_QMH_Enqueue Message (poly).vi"("Message"="Configuration dialog", "Message Queue in"=w541) -> ("error out"=w542:errorcluster)  [unwired: 8 in, 1 out]
          }
          event Value Change {
            n206 = event-data() -> ()  [unwired: 1 in, 1 out]
            n207 = call-poly <vilib>:"Delacor_lib_QMH_Enqueue Message (poly).vi"("Message"="Move motor", "Message Queue in"=w544) -> ("error out"=w545:errorcluster)  [unwired: 8 in, 1 out]
          }
          event User Event {
            # "Another Module called the \"Start motor\" API Method."
            n208 = event-data() -> ("Motor params"=w547:T23)  [unwired: 1 in]
            n209 = Bundle(cluster=T22 {"Motor params"={"Dirección"=enum."Avance", "Tipo"=enum."Simple", "Velocidad (RPM)"=5.0, "Cantidad de pasos"=1, "Avance (mm)"=0.0, "Pasos por rev"=200.0, "Paso del tonillo"=0.0}} ("Start motor Argument"), "Motor params"=w547) -> (w548:T22)
            n210 = call-poly <vilib>:"Delacor_lib_QMH_Enqueue Message (poly).vi"("Message Data"=w548, "Message"="Start motor", "Message Queue in"=w551) -> ("error out"=w546:errorcluster)  [unwired: 7 in, 1 out]
          }
          event User Event {
            # "Show the panel of this VI, and send a status updated message to let listeners know."
            # "Another Module called the \"Show Panel\" API Method."
            n211 = event-data() -> ()  [unwired: 1 in, 1 out]
            n212 = control-ref of="This VI"() -> (w553:refnum<vi>)
            n213 = call "Open VI Panel.vi"("VI"=w553) -> ()  [unwired: 10 in, 1 out]
            n214 = call "Status Updated.vi"("Status"="Panel shown." ("format string")) -> ()  [unwired: 10 in, 1 out]
          }
          event User Event {
            # "Hide the panel of this VI, and send a status updated message to let listeners know."
            # "Another Module called the \"Hide Panel\" API Method."
            n215 = event-data() -> ()  [unwired: 1 in, 1 out]
            n216 = control-ref of="This VI"() -> (w555:refnum<vi>)
            n217 = call "Hide VI Panel.vi"("VI"=w555) -> ()  [unwired: 10 in, 1 out]
            n218 = call "Status Updated.vi"("Status"="Panel hidden." ("format string")) -> ()  [unwired: 10 in, 1 out]
          }
          event User Event {
            # "Another Module called the \"Get Module Execution Status\" API Method."
            n219 = event-data() -> ()  [unwired: 1 in, 1 out]
            n220 = call "Update Module Execution Status.vi"("Running?"=TRUE) -> ("error out"=w557:errorcluster)  [unwired: 10 in]
          }
          event User Event {
            # "Another Module called the \"Show Diagram\" API Method. This event is used for debugging."
            n221 = event-data() -> ()  [unwired: 1 in, 1 out]
            n222 = disable-structure shown="RUN_TIME_ENGINE==False" {
              frame condition #0 (active) {
                # "functionality not available in exe"
                n223 = invoke class="VI" method="Lock State.Get"() -> (error out=w563:errorcluster, "Get Lock State"=w562:T27, "pwd in cache"=w559:bool)  [unwired: 4 in, 1 out]
                n224 = Equal?(x=T27."Password-protected", y=w562) -> (x = y?=w560:bool)
                n225 = Compound Arithmetic op=AND(w560, invert w559) -> (w558:bool)
                n226 = case shown="False" w558 {
                  tunnel: w563 -> [w566 _]
                  frame False {
                    n227 = property class="VI"(error in=w566, "BDWin.Open"=TRUE ("Block Diagram Window:Open")) -> ()  [unwired: 1 in, 2 out]
                    n228 = call "Status Updated.vi"("Status"="Block Diagram shown." ("format string")) -> ()  [unwired: 10 in, 1 out]
                  }
                  frame True {
                    # "Password-protected VI, and the password is not in the cache. Do not show the diagram."
                  }
                }
              }
              frame condition #1 {
              }
            }
          }
          event User Event {
            # "The Stop Module Event can get fired from the Exit message in the MHL. The queue gets destroyed in that case. If the queue no longer exists, the Enqueue Exit as a priority message will return error 1. It is safe to ignore, because the module is already exiting."
            # "Another Module called the \"Stop Module\" API Method  or the Message Handling Loop below."
            n229 = event-data() -> ("Origin"=w573:string, "Exit via Stop Module Req?"=w569:bool, "Wait for Module to stop?"=w568:bool)  [unwired: 1 in]
            n230 = local write "Status"(w573) -> ()
            n231 = Bundle By Name(cluster=T26 {"Origin"="", "Exit via Stop Module Req?"=FALSE, "Wait for Module to stop?"=FALSE} ("Stop Argument"), "Exit via Stop Module Req?"=w569, "Wait for Module to stop?"=w568) -> (w567:T26)
            n232 = call-poly <vilib>:"Delacor_lib_QMH_Enqueue Message (poly).vi"("Priority Message? (F)"=TRUE, "Message Data"=w567, "Message"="Exit", "Message Queue in"=w574) -> ("error out"=w578:errorcluster)  [unwired: 6 in, 1 out]
            n233 = call <vilib>:"Clear Errors.vi"("error in (no error)"=w578, "specific error code to clear (0: all)"=1) -> ("error out"=w577:errorcluster)  [unwired: 4 in, 1 out]
          }
          event User Event {
            n234 = event-data() -> ("Stop condition"=w579:string)  [unwired: 1 in]
            n235 = call-poly <vilib>:"Delacor_lib_QMH_Enqueue Message (poly).vi"("Message Data"=w579, "Message"="Update status", "Message Queue in"=w581) -> ("error out"=w582:errorcluster)  [unwired: 7 in, 1 out]
          }
          event Panel Close? {
            w586 = TRUE  # Discard the event, the MHL is responsible for closing and stopping this VI.
            # "Hide the panel or send the 'Exit' message if the user clicks the 'X' on the module main VI panel."
            n236 = event-data() -> ()  [unwired: 1 in, 1 out]
            n237 = property class="Module Admin"(reference=w584) -> ("Accessors:External Launch"=w583:bool)  [unwired: 1 in, 2 out]
            n238 = case shown="False" w583 {
              tunnel: w585 -> [_ w591]
              tunnel: [_ w592] -> w587
              frame True {
                # "If externally launched, clicking the 'X' hides the panel, but doesn't close it."
                n239 = control-ref of="This VI"() -> (w588:refnum<vi>)
                n240 = call "Hide VI Panel.vi"("VI"=w588) -> ()  [unwired: 10 in, 1 out]
              }
              frame False {
                # "If run as a stand-alone VI, clicking the panel 'X' stops the VI."
                n241 = call-poly <vilib>:"Delacor_lib_QMH_Enqueue Message (poly).vi"("Priority Message? (F)"=TRUE, "Message"="Exit", "Message Queue in"=w591) -> ("error out"=w592:errorcluster)  [unwired: 7 in, 1 out]
              }
            }
            n242 = event-data("Discard?"=w586) -> ()  [unwired: 1 in, 1 out]
          }
          event Value Change {
            n243 = event-data() -> ()  [unwired: 1 in, 1 out]
            n244 = call-poly <vilib>:"Delacor_lib_QMH_Enqueue Message (poly).vi"("Message"="Home", "Message Queue in"=w594) -> ("error out"=w595:errorcluster)  [unwired: 8 in, 1 out]
          }
          event Value Change {
            n245 = event-data() -> ("NewVal"=w596:T1)  [unwired: 1 in]
            n246 = call-poly <vilib>:"Delacor_lib_QMH_Enqueue Message (poly).vi"("Message Data"=w596, "Message"="Stop motor", "Message Queue in"=w598) -> ("error out"=w599:errorcluster)  [unwired: 7 in, 1 out]
          }
          event Value Change {
            n247 = event-data() -> ()  [unwired: 1 in, 1 out]
            n248 = call-poly <vilib>:"Delacor_lib_QMH_Enqueue Message (poly).vi"("Message"="Exit", "Message Queue in"=w601) -> ("error out"=w602:errorcluster)  [unwired: 8 in, 1 out]
          }
        }
        n249 = call-dynamic "Delacor_lib_QMH_Error Handler - Event Handling Loop.vi"("error in"=w508, "Message Queue in"=w502) -> ("dup error in"=w507:errorcluster)  [unwired: 8 in, 1 out]
      }
    }
    frame Error {
      # "Synchronize Caller Events.vi will inform Start Module.vi that the module has launched and will let the code calling Start Module.vi register for broadcasts and would permit the caller receive the broadcast that an error occurred at launch time."
      n250 = Unbundle By Name(w604) -> ("DAQ mod ID"=w603:i32)
      n251 = call-dynamic "Delacor_lib_QMH_Release Message Queue.vi"("error in"=w609, "Message Queue"=w607) -> ("error out"=w608:errorcluster)  [unwired: 9 in]
      n252 = call "Synchronize Caller Events.vi"("Singleton Module Admin in"=w610) -> ("error out"=w615:errorcluster)  [unwired: 9 in, 1 out]
      n253 = call "Module Name--constant.vi"() -> ("Module Name"=w613:string)  [unwired: 11 in]
      n254 = Format Into String(format string="An error occurred during initialization. %s is no longer running.", w613) -> (resulting string=w611:string)  [unwired: 2 in, 1 out]
      n255 = Merge Errors(w608, w615) -> (w616:errorcluster)
      n256 = call "Stop Module.vi"("Module ID"=-1) -> ()  [unwired: 10 in, 1 out]
      n257 = call "Stop Module.vi"("Module ID"=w603) -> ()  [unwired: 10 in, 1 out]
      n258 = call "Stop Module.vi"() -> ()  [unwired: 11 in, 1 out]
      n259 = call "Error Reported.vi"("Additional Information"=w611, "Error"=w616) -> ()  [unwired: 9 in, 1 out]
    }
  }
  n260 = Merge Errors(w34, w37) -> (w33:errorcluster)
  n261 = call "Close Module.vi"("error in (no error)"=w33, "Module Admin in"=w22) -> ("error out"=w35:errorcluster, "External Launch"=w25:bool, "Module Admin out"=w26:refnum<class "Delacor_lib_QMH_Module Admin.lvclass">)  [unwired: 7 in]
  n262 = Unregister For Events(event registration refnum=w30, error in=w35) -> (error out=w21:errorcluster)
  n263 = Unregister For Events(event registration refnum=w19, error in=w21) -> (error out=w20:errorcluster)
  "error out" <- w20
  n264 = local write "Module Admin"(w26) -> ()
  n265 = disable-structure shown="Default" {
    disable-tunnel: w25 -> [w618 _]
    disable-tunnel: w20 -> [w617 _]
    frame condition #0 (active) {
      n266 = case "External Launch?" shown="False" w618 {
        tunnel: w617 -> [_ w619]
        frame False {
        }
        frame True {
          n267 = case shown="No Error" w619 {
            frame No Error {
              n268 = invoke on="Invoke Node" class="VI" method="FP.Close"() -> ()  [unwired: 3 in, 3 out]
            }
            frame Error {
              n269 = invoke on="Invoke Node" class="VI" method="FP.Open"("Activate"=TRUE ("Activate?")) -> ()  [unwired: 4 in, 5 out]
            }
          }
        }
      }
    }
    frame condition #1 {
      n270 = Quit LabVIEW() -> ()  [unwired: 1 in]
    }
  }
